vi "Field vs  IV and Ic distribution_V2.vi"() -> ()   [LabVIEW 2020]
uses:
  RT fast data.ctl
  <vilib>/LabVIEW Targets/FPGA/cRIO/shared/nicrio_ModuleControls/nicrio_cRIO-9775_RecordDataRates4ChansRing.ctl
  <vilib>/Utility/file.llb/Write Delimited Spreadsheet (DBL).vi
  global.vi
  <resource>/objmgr/ni.dex.rc
  <vilib>/Analysis/NI_AALBase.lvlib
panel:
  in  "Tab Control":enum32{"Field", "cRIO", "IV Ic Parameters"}(tab)=enum."cRIO"
  in  "Field Rate mT per sec":dbl=0.1 format="%#_13g"
  in  "Field Radius mT":dbl=10.0 format="%#_13g"
  in  "Field step mT":dbl=0.05 format="%#_13g"
  in  "Field Origin mT":dbl=-6.0 format="%#_13g"
  in  "Ramp up first T":bool=TRUE
  in  "Ramp type":string(combo)="Range"
  in  "Magnet Device Select":string(combo)="Elsa Magnet mT"
  in  "AI Channel":u8
  in  "Trigger Slope":enum8{"Positive", "Negative"}(ring)
  in  "Dist Record Samples":u32=10000
  in  "cRIO IP":string="//172.22.11.2"
  in  "Data buffer size":i32=1000
  in  "Voltage Scale factor":dbl=0.0001
  in  "Current Scale factor":dbl=1.0
  in  "IV Record Samples":u32=5000
  in  "Gate wait time us":u32=150
  in  "IV Record Data Rate":T1=200 items=["20.000 MS/s (NI 9775)"=1, "10.00 MS/s (NI 9775)"=2, "6.667 MS/s (NI 9775)"=3, "5.000 MS/s (NI 9775)"=4, "2.500 MS/s (NI 9775)"=8, "1.667 MS/s (NI 9775)"=12, "1.250 MS/s (NI 9775)"=16, "1.000 MS/s (NI 9775)"=20, "833.333 KS/s (NI 9775)"=24, "714.286 KS/s (NI 9775)"=28, "625.000 KS/s (NI 9775)"=32, "555.556 KS/s (NI 9775)"=36, "500.000 KS/s (NI 9775)"=40, "454.545 KS/s (NI 9775)"=44, "416.667 KS/s (NI 9775)"=48, "384.615 KS/s (NI 9775)"=52, "357.143 KS/s (NI 9775)"=56, "333.333 KS/s (NI 9775)"=60, "312.500 KS/s (NI 9775)"=64, "294.118 KS/s (NI 9775)"=68, "277.778 KS/s (NI 9775)"=72, "263.158 KS/s (NI 9775)"=76, "250.000 KS/s (NI 9775)"=80, "238.095 KS/s (NI 9775)"=84, "227.273 KS/s (NI 9775)"=88, "217.391 KS/s (NI 9775)"=92, "208.333 KS/s (NI 9775)"=96, "200.000 KS/s (NI 9775)"=100, "192.308 KS/s (NI 9775)"=104, "185.185 KS/s (NI 9775)"=108, "178.571 KS/s (NI 9775)"=112, "172.414 KS/s (NI 9775)"=116, "166.667 KS/s (NI 9775)"=120, "161.290 KS/s (NI 9775)"=124, "156.250 KS/s (NI 9775)"=128, "151.515 KS/s (NI 9775)"=132, "147.059 KS/s (NI 9775)"=136, "142.857 KS/s (NI 9775)"=140, "138.889 KS/s (NI 9775)"=144, "135.135 KS/s (NI 9775)"=148, "131.579 KS/s (NI 9775)"=152, "128.205 KS/s (NI 9775)"=156, "125.000 KS/s (NI 9775)"=160, "121.951 KS/s (NI 9775)"=164, "119.048 KS/s (NI 9775)"=168, "116.279 KS/s (NI 9775)"=172, "113.636 KS/s (NI 9775)"=176, "111.111 KS/s (NI 9775)"=180, "108.696 KS/s (NI 9775)"=184, "106.383 KS/s (NI 9775)"=188, "104.167 KS/s (NI 9775)"=192, "102.041 KS/s (NI 9775)"=196, "100.000 KS/s (NI 9775)"=200, "50.000 KS/s (NI 9775)"=400, "33.333 KS/s (NI 9775)"=600, "25.000 KS/s (NI 9775)"=800, "20.000 KS/s (NI 9775)"=1000, "16.667 KS/s (NI 9775)"=1200, "14.286 KS/s (NI 9775)"=1400, "12.500 KS/s (NI 9775)"=1600, "11.111 KS/s (NI 9775)"=1800, "10.000 KS/s (NI 9775)"=2000, "9.091 KS/s (NI 9775)"=2200, "8.333 KS/s (NI 9775)"=2400, "7.692 KS/s (NI 9775)"=2600, "7.143 KS/s (NI 9775)"=2800, "6.667 KS/s (NI 9775)"=3000, "6.250 KS/s (NI 9775)"=3200, "5.882 KS/s (NI 9775)"=3400, "5.556 KS/s (NI 9775)"=3600, "5.000 KS/s (NI 9775)"=4000, "4.762 KS/s (NI 9775)"=4200, "4.545 KS/s (NI 9775)"=4400, "4.348 KS/s (NI 9775)"=4600, "4.167 KS/s (NI 9775)"=4800, "4.000 KS/s (NI 9775)"=5000, "3.846 KS/s (NI 9775)"=5200, "3.571 KS/s (NI 9775)"=5600, "3.333 KS/s (NI 9775)"=6000, "3.125 KS/s (NI 9775)"=6400, "2.941 KS/s (NI 9775)"=6800, "2.778 KS/s (NI 9775)"=7200, "2.632 KS/s (NI 9775)"=7600, "2.500 KS/s (NI 9775)"=8000, "2.381 KS/s (NI 9775)"=8400, "2.273 KS/s (NI 9775)"=8800, "2.174 KS/s (NI 9775)"=9200, "2.083 KS/s (NI 9775)"=9600, "2.000 KS/s (NI 9775)"=10000, "1.923 KS/s (NI 9775)"=10400, "1.852 KS/s (NI 9775)"=10800, "1.786 KS/s (NI 9775)"=11200, "1.724 KS/s (NI 9775)"=11600, "1.667 KS/s (NI 9775)"=12000, "1.613 KS/s (NI 9775)"=12400, "1.563 KS/s (NI 9775)"=12800, "1.515 KS/s (NI 9775)"=13200, "1.471 KS/s (NI 9775)"=13600, "1.429 KS/s (NI 9775)"=14000, "1.389 KS/s (NI 9775)"=14400, "1.351 KS/s (NI 9775)"=14800, "1.316 KS/s (NI 9775)"=15200, "1.282 KS/s (NI 9775)"=15600, "1.250 KS/s (NI 9775)"=16000, "1.220 KS/s (NI 9775)"=16400, "1.190 KS/s (NI 9775)"=16800, "1.163 KS/s (NI 9775)"=17200, "1.136 KS/s (NI 9775)"=17600, "1.111 KS/s (NI 9775)"=18000, "1.087 KS/s (NI 9775)"=18400, "1.064 KS/s (NI 9775)"=18800, "1.042 KS/s (NI 9775)"=19200, "1.020 KS/s (NI 9775)"=19600, "1.000 KS/s (NI 9775)"=20000, "0.980 KS/s (NI 9775)"=20400, "0.962 KS/s (NI 9775)"=20800, "0.943 KS/s (NI 9775)"=21200, "0.926 KS/s (NI 9775)"=21600, "0.909 KS/s (NI 9775)"=22000, "0.893 KS/s (NI 9775)"=22400, "0.877 KS/s (NI 9775)"=22800, "0.862 KS/s (NI 9775)"=23200, "0.847 KS/s (NI 9775)"=23600, "0.833 KS/s (NI 9775)"=24000, "0.820 KS/s (NI 9775)"=24400, "0.806 KS/s (NI 9775)"=24800, "0.794 KS/s (NI 9775)"=25200, "0.781 KS/s (NI 9775)"=25600, "0.694 KS/s (NI 9775)"=28800, "0.625 KS/s (NI 9775)"=32000, "0.568 KS/s (NI 9775)"=35200, "0.521 KS/s (NI 9775)"=38400, "0.446 KS/s (NI 9775)"=44800, "0.391 KS/s (NI 9775)"=51200, "0.347 KS/s (NI 9775)"=57600, "0.313 KS/s (NI 9775)"=64000]
  in  "Relative threshold":dbl=0.21 format="%#_13g"
  in  "Dist Record Data Rate":T1=1 items=["20.000 MS/s (NI 9775)"=1, "10.00 MS/s (NI 9775)"=2, "6.667 MS/s (NI 9775)"=3, "5.000 MS/s (NI 9775)"=4, "2.500 MS/s (NI 9775)"=8, "1.667 MS/s (NI 9775)"=12, "1.250 MS/s (NI 9775)"=16, "1.000 MS/s (NI 9775)"=20, "833.333 KS/s (NI 9775)"=24, "714.286 KS/s (NI 9775)"=28, "625.000 KS/s (NI 9775)"=32, "555.556 KS/s (NI 9775)"=36, "500.000 KS/s (NI 9775)"=40, "454.545 KS/s (NI 9775)"=44, "416.667 KS/s (NI 9775)"=48, "384.615 KS/s (NI 9775)"=52, "357.143 KS/s (NI 9775)"=56, "333.333 KS/s (NI 9775)"=60, "312.500 KS/s (NI 9775)"=64, "294.118 KS/s (NI 9775)"=68, "277.778 KS/s (NI 9775)"=72, "263.158 KS/s (NI 9775)"=76, "250.000 KS/s (NI 9775)"=80, "238.095 KS/s (NI 9775)"=84, "227.273 KS/s (NI 9775)"=88, "217.391 KS/s (NI 9775)"=92, "208.333 KS/s (NI 9775)"=96, "200.000 KS/s (NI 9775)"=100, "192.308 KS/s (NI 9775)"=104, "185.185 KS/s (NI 9775)"=108, "178.571 KS/s (NI 9775)"=112, "172.414 KS/s (NI 9775)"=116, "166.667 KS/s (NI 9775)"=120, "161.290 KS/s (NI 9775)"=124, "156.250 KS/s (NI 9775)"=128, "151.515 KS/s (NI 9775)"=132, "147.059 KS/s (NI 9775)"=136, "142.857 KS/s (NI 9775)"=140, "138.889 KS/s (NI 9775)"=144, "135.135 KS/s (NI 9775)"=148, "131.579 KS/s (NI 9775)"=152, "128.205 KS/s (NI 9775)"=156, "125.000 KS/s (NI 9775)"=160, "121.951 KS/s (NI 9775)"=164, "119.048 KS/s (NI 9775)"=168, "116.279 KS/s (NI 9775)"=172, "113.636 KS/s (NI 9775)"=176, "111.111 KS/s (NI 9775)"=180, "108.696 KS/s (NI 9775)"=184, "106.383 KS/s (NI 9775)"=188, "104.167 KS/s (NI 9775)"=192, "102.041 KS/s (NI 9775)"=196, "100.000 KS/s (NI 9775)"=200, "50.000 KS/s (NI 9775)"=400, "33.333 KS/s (NI 9775)"=600, "25.000 KS/s (NI 9775)"=800, "20.000 KS/s (NI 9775)"=1000, "16.667 KS/s (NI 9775)"=1200, "14.286 KS/s (NI 9775)"=1400, "12.500 KS/s (NI 9775)"=1600, "11.111 KS/s (NI 9775)"=1800, "10.000 KS/s (NI 9775)"=2000, "9.091 KS/s (NI 9775)"=2200, "8.333 KS/s (NI 9775)"=2400, "7.692 KS/s (NI 9775)"=2600, "7.143 KS/s (NI 9775)"=2800, "6.667 KS/s (NI 9775)"=3000, "6.250 KS/s (NI 9775)"=3200, "5.882 KS/s (NI 9775)"=3400, "5.556 KS/s (NI 9775)"=3600, "5.000 KS/s (NI 9775)"=4000, "4.762 KS/s (NI 9775)"=4200, "4.545 KS/s (NI 9775)"=4400, "4.348 KS/s (NI 9775)"=4600, "4.167 KS/s (NI 9775)"=4800, "4.000 KS/s (NI 9775)"=5000, "3.846 KS/s (NI 9775)"=5200, "3.571 KS/s (NI 9775)"=5600, "3.333 KS/s (NI 9775)"=6000, "3.125 KS/s (NI 9775)"=6400, "2.941 KS/s (NI 9775)"=6800, "2.778 KS/s (NI 9775)"=7200, "2.632 KS/s (NI 9775)"=7600, "2.500 KS/s (NI 9775)"=8000, "2.381 KS/s (NI 9775)"=8400, "2.273 KS/s (NI 9775)"=8800, "2.174 KS/s (NI 9775)"=9200, "2.083 KS/s (NI 9775)"=9600, "2.000 KS/s (NI 9775)"=10000, "1.923 KS/s (NI 9775)"=10400, "1.852 KS/s (NI 9775)"=10800, "1.786 KS/s (NI 9775)"=11200, "1.724 KS/s (NI 9775)"=11600, "1.667 KS/s (NI 9775)"=12000, "1.613 KS/s (NI 9775)"=12400, "1.563 KS/s (NI 9775)"=12800, "1.515 KS/s (NI 9775)"=13200, "1.471 KS/s (NI 9775)"=13600, "1.429 KS/s (NI 9775)"=14000, "1.389 KS/s (NI 9775)"=14400, "1.351 KS/s (NI 9775)"=14800, "1.316 KS/s (NI 9775)"=15200, "1.282 KS/s (NI 9775)"=15600, "1.250 KS/s (NI 9775)"=16000, "1.220 KS/s (NI 9775)"=16400, "1.190 KS/s (NI 9775)"=16800, "1.163 KS/s (NI 9775)"=17200, "1.136 KS/s (NI 9775)"=17600, "1.111 KS/s (NI 9775)"=18000, "1.087 KS/s (NI 9775)"=18400, "1.064 KS/s (NI 9775)"=18800, "1.042 KS/s (NI 9775)"=19200, "1.020 KS/s (NI 9775)"=19600, "1.000 KS/s (NI 9775)"=20000, "0.980 KS/s (NI 9775)"=20400, "0.962 KS/s (NI 9775)"=20800, "0.943 KS/s (NI 9775)"=21200, "0.926 KS/s (NI 9775)"=21600, "0.909 KS/s (NI 9775)"=22000, "0.893 KS/s (NI 9775)"=22400, "0.877 KS/s (NI 9775)"=22800, "0.862 KS/s (NI 9775)"=23200, "0.847 KS/s (NI 9775)"=23600, "0.833 KS/s (NI 9775)"=24000, "0.820 KS/s (NI 9775)"=24400, "0.806 KS/s (NI 9775)"=24800, "0.794 KS/s (NI 9775)"=25200, "0.781 KS/s (NI 9775)"=25600, "0.694 KS/s (NI 9775)"=28800, "0.625 KS/s (NI 9775)"=32000, "0.568 KS/s (NI 9775)"=35200, "0.521 KS/s (NI 9775)"=38400, "0.446 KS/s (NI 9775)"=44800, "0.391 KS/s (NI 9775)"=51200, "0.347 KS/s (NI 9775)"=57600, "0.313 KS/s (NI 9775)"=64000]
  in  "Zero avg":i32=500
  in  "Count ms half of T":u32=15
  in  "Wait before trigger us":u32=10100
  in  "Tab Control 2":enum32{"IV", "Ic"}(tab)
  out "IV parameters":T2={"Records Num"=1, "AI Trigger Configuration"={"Trigger Slope"=enum."Positive", "Trigger Level"=0.10009765625, "Hystesis Value"=0.094970703125, "AI Channel"=0}, "Record PreTrigger Samples"=1, "Record Samples"=5000, "Ic Cut off or curve"=FALSE, "Gate wait time us"=150, "Record Data Rate"=200, "Count ms half of T"=15, "Wait before trigger us"=10100} {"Record Data Rate" items=["20.000 MS/s (NI 9775)"=1, "10.00 MS/s (NI 9775)"=2, "6.667 MS/s (NI 9775)"=3, "5.000 MS/s (NI 9775)"=4, "2.500 MS/s (NI 9775)"=8, "1.667 MS/s (NI 9775)"=12, "1.250 MS/s (NI 9775)"=16, "1.000 MS/s (NI 9775)"=20, "833.333 KS/s (NI 9775)"=24, "714.286 KS/s (NI 9775)"=28, "625.000 KS/s (NI 9775)"=32, "555.556 KS/s (NI 9775)"=36, "500.000 KS/s (NI 9775)"=40, "454.545 KS/s (NI 9775)"=44, "416.667 KS/s (NI 9775)"=48, "384.615 KS/s (NI 9775)"=52, "357.143 KS/s (NI 9775)"=56, "333.333 KS/s (NI 9775)"=60, "312.500 KS/s (NI 9775)"=64, "294.118 KS/s (NI 9775)"=68, "277.778 KS/s (NI 9775)"=72, "263.158 KS/s (NI 9775)"=76, "250.000 KS/s (NI 9775)"=80, "238.095 KS/s (NI 9775)"=84, "227.273 KS/s (NI 9775)"=88, "217.391 KS/s (NI 9775)"=92, "208.333 KS/s (NI 9775)"=96, "200.000 KS/s (NI 9775)"=100, "192.308 KS/s (NI 9775)"=104, "185.185 KS/s (NI 9775)"=108, "178.571 KS/s (NI 9775)"=112, "172.414 KS/s (NI 9775)"=116, "166.667 KS/s (NI 9775)"=120, "161.290 KS/s (NI 9775)"=124, "156.250 KS/s (NI 9775)"=128, "151.515 KS/s (NI 9775)"=132, "147.059 KS/s (NI 9775)"=136, "142.857 KS/s (NI 9775)"=140, "138.889 KS/s (NI 9775)"=144, "135.135 KS/s (NI 9775)"=148, "131.579 KS/s (NI 9775)"=152, "128.205 KS/s (NI 9775)"=156, "125.000 KS/s (NI 9775)"=160, "121.951 KS/s (NI 9775)"=164, "119.048 KS/s (NI 9775)"=168, "116.279 KS/s (NI 9775)"=172, "113.636 KS/s (NI 9775)"=176, "111.111 KS/s (NI 9775)"=180, "108.696 KS/s (NI 9775)"=184, "106.383 KS/s (NI 9775)"=188, "104.167 KS/s (NI 9775)"=192, "102.041 KS/s (NI 9775)"=196, "100.000 KS/s (NI 9775)"=200, "50.000 KS/s (NI 9775)"=400, "33.333 KS/s (NI 9775)"=600, "25.000 KS/s (NI 9775)"=800, "20.000 KS/s (NI 9775)"=1000, "16.667 KS/s (NI 9775)"=1200, "14.286 KS/s (NI 9775)"=1400, "12.500 KS/s (NI 9775)"=1600, "11.111 KS/s (NI 9775)"=1800, "10.000 KS/s (NI 9775)"=2000, "9.091 KS/s (NI 9775)"=2200, "8.333 KS/s (NI 9775)"=2400, "7.692 KS/s (NI 9775)"=2600, "7.143 KS/s (NI 9775)"=2800, "6.667 KS/s (NI 9775)"=3000, "6.250 KS/s (NI 9775)"=3200, "5.882 KS/s (NI 9775)"=3400, "5.556 KS/s (NI 9775)"=3600, "5.000 KS/s (NI 9775)"=4000, "4.762 KS/s (NI 9775)"=4200, "4.545 KS/s (NI 9775)"=4400, "4.348 KS/s (NI 9775)"=4600, "4.167 KS/s (NI 9775)"=4800, "4.000 KS/s (NI 9775)"=5000, "3.846 KS/s (NI 9775)"=5200, "3.571 KS/s (NI 9775)"=5600, "3.333 KS/s (NI 9775)"=6000, "3.125 KS/s (NI 9775)"=6400, "2.941 KS/s (NI 9775)"=6800, "2.778 KS/s (NI 9775)"=7200, "2.632 KS/s (NI 9775)"=7600, "2.500 KS/s (NI 9775)"=8000, "2.381 KS/s (NI 9775)"=8400, "2.273 KS/s (NI 9775)"=8800, "2.174 KS/s (NI 9775)"=9200, "2.083 KS/s (NI 9775)"=9600, "2.000 KS/s (NI 9775)"=10000, "1.923 KS/s (NI 9775)"=10400, "1.852 KS/s (NI 9775)"=10800, "1.786 KS/s (NI 9775)"=11200, "1.724 KS/s (NI 9775)"=11600, "1.667 KS/s (NI 9775)"=12000, "1.613 KS/s (NI 9775)"=12400, "1.563 KS/s (NI 9775)"=12800, "1.515 KS/s (NI 9775)"=13200, "1.471 KS/s (NI 9775)"=13600, "1.429 KS/s (NI 9775)"=14000, "1.389 KS/s (NI 9775)"=14400, "1.351 KS/s (NI 9775)"=14800, "1.316 KS/s (NI 9775)"=15200, "1.282 KS/s (NI 9775)"=15600, "1.250 KS/s (NI 9775)"=16000, "1.220 KS/s (NI 9775)"=16400, "1.190 KS/s (NI 9775)"=16800, "1.163 KS/s (NI 9775)"=17200, "1.136 KS/s (NI 9775)"=17600, "1.111 KS/s (NI 9775)"=18000, "1.087 KS/s (NI 9775)"=18400, "1.064 KS/s (NI 9775)"=18800, "1.042 KS/s (NI 9775)"=19200, "1.020 KS/s (NI 9775)"=19600, "1.000 KS/s (NI 9775)"=20000, "0.980 KS/s (NI 9775)"=20400, "0.962 KS/s (NI 9775)"=20800, "0.943 KS/s (NI 9775)"=21200, "0.926 KS/s (NI 9775)"=21600, "0.909 KS/s (NI 9775)"=22000, "0.893 KS/s (NI 9775)"=22400, "0.877 KS/s (NI 9775)"=22800, "0.862 KS/s (NI 9775)"=23200, "0.847 KS/s (NI 9775)"=23600, "0.833 KS/s (NI 9775)"=24000, "0.820 KS/s (NI 9775)"=24400, "0.806 KS/s (NI 9775)"=24800, "0.794 KS/s (NI 9775)"=25200, "0.781 KS/s (NI 9775)"=25600, "0.694 KS/s (NI 9775)"=28800, "0.625 KS/s (NI 9775)"=32000, "0.568 KS/s (NI 9775)"=35200, "0.521 KS/s (NI 9775)"=38400, "0.446 KS/s (NI 9775)"=44800, "0.391 KS/s (NI 9775)"=51200, "0.347 KS/s (NI 9775)"=57600, "0.313 KS/s (NI 9775)"=64000]}
  out "Ic parameters":T2={"Records Num"=10000, "AI Trigger Configuration"={"Trigger Slope"=enum."Positive", "Trigger Level"=0.2392578125, "Hystesis Value"=0.0, "AI Channel"=0}, "Record PreTrigger Samples"=1, "Record Samples"=16, "Ic Cut off or curve"=TRUE, "Gate wait time us"=150, "Record Data Rate"=1, "Count ms half of T"=15, "Wait before trigger us"=10100} {"Record Data Rate" items=["20.000 MS/s (NI 9775)"=1, "10.00 MS/s (NI 9775)"=2, "6.667 MS/s (NI 9775)"=3, "5.000 MS/s (NI 9775)"=4, "2.500 MS/s (NI 9775)"=8, "1.667 MS/s (NI 9775)"=12, "1.250 MS/s (NI 9775)"=16, "1.000 MS/s (NI 9775)"=20, "833.333 KS/s (NI 9775)"=24, "714.286 KS/s (NI 9775)"=28, "625.000 KS/s (NI 9775)"=32, "555.556 KS/s (NI 9775)"=36, "500.000 KS/s (NI 9775)"=40, "454.545 KS/s (NI 9775)"=44, "416.667 KS/s (NI 9775)"=48, "384.615 KS/s (NI 9775)"=52, "357.143 KS/s (NI 9775)"=56, "333.333 KS/s (NI 9775)"=60, "312.500 KS/s (NI 9775)"=64, "294.118 KS/s (NI 9775)"=68, "277.778 KS/s (NI 9775)"=72, "263.158 KS/s (NI 9775)"=76, "250.000 KS/s (NI 9775)"=80, "238.095 KS/s (NI 9775)"=84, "227.273 KS/s (NI 9775)"=88, "217.391 KS/s (NI 9775)"=92, "208.333 KS/s (NI 9775)"=96, "200.000 KS/s (NI 9775)"=100, "192.308 KS/s (NI 9775)"=104, "185.185 KS/s (NI 9775)"=108, "178.571 KS/s (NI 9775)"=112, "172.414 KS/s (NI 9775)"=116, "166.667 KS/s (NI 9775)"=120, "161.290 KS/s (NI 9775)"=124, "156.250 KS/s (NI 9775)"=128, "151.515 KS/s (NI 9775)"=132, "147.059 KS/s (NI 9775)"=136, "142.857 KS/s (NI 9775)"=140, "138.889 KS/s (NI 9775)"=144, "135.135 KS/s (NI 9775)"=148, "131.579 KS/s (NI 9775)"=152, "128.205 KS/s (NI 9775)"=156, "125.000 KS/s (NI 9775)"=160, "121.951 KS/s (NI 9775)"=164, "119.048 KS/s (NI 9775)"=168, "116.279 KS/s (NI 9775)"=172, "113.636 KS/s (NI 9775)"=176, "111.111 KS/s (NI 9775)"=180, "108.696 KS/s (NI 9775)"=184, "106.383 KS/s (NI 9775)"=188, "104.167 KS/s (NI 9775)"=192, "102.041 KS/s (NI 9775)"=196, "100.000 KS/s (NI 9775)"=200, "50.000 KS/s (NI 9775)"=400, "33.333 KS/s (NI 9775)"=600, "25.000 KS/s (NI 9775)"=800, "20.000 KS/s (NI 9775)"=1000, "16.667 KS/s (NI 9775)"=1200, "14.286 KS/s (NI 9775)"=1400, "12.500 KS/s (NI 9775)"=1600, "11.111 KS/s (NI 9775)"=1800, "10.000 KS/s (NI 9775)"=2000, "9.091 KS/s (NI 9775)"=2200, "8.333 KS/s (NI 9775)"=2400, "7.692 KS/s (NI 9775)"=2600, "7.143 KS/s (NI 9775)"=2800, "6.667 KS/s (NI 9775)"=3000, "6.250 KS/s (NI 9775)"=3200, "5.882 KS/s (NI 9775)"=3400, "5.556 KS/s (NI 9775)"=3600, "5.000 KS/s (NI 9775)"=4000, "4.762 KS/s (NI 9775)"=4200, "4.545 KS/s (NI 9775)"=4400, "4.348 KS/s (NI 9775)"=4600, "4.167 KS/s (NI 9775)"=4800, "4.000 KS/s (NI 9775)"=5000, "3.846 KS/s (NI 9775)"=5200, "3.571 KS/s (NI 9775)"=5600, "3.333 KS/s (NI 9775)"=6000, "3.125 KS/s (NI 9775)"=6400, "2.941 KS/s (NI 9775)"=6800, "2.778 KS/s (NI 9775)"=7200, "2.632 KS/s (NI 9775)"=7600, "2.500 KS/s (NI 9775)"=8000, "2.381 KS/s (NI 9775)"=8400, "2.273 KS/s (NI 9775)"=8800, "2.174 KS/s (NI 9775)"=9200, "2.083 KS/s (NI 9775)"=9600, "2.000 KS/s (NI 9775)"=10000, "1.923 KS/s (NI 9775)"=10400, "1.852 KS/s (NI 9775)"=10800, "1.786 KS/s (NI 9775)"=11200, "1.724 KS/s (NI 9775)"=11600, "1.667 KS/s (NI 9775)"=12000, "1.613 KS/s (NI 9775)"=12400, "1.563 KS/s (NI 9775)"=12800, "1.515 KS/s (NI 9775)"=13200, "1.471 KS/s (NI 9775)"=13600, "1.429 KS/s (NI 9775)"=14000, "1.389 KS/s (NI 9775)"=14400, "1.351 KS/s (NI 9775)"=14800, "1.316 KS/s (NI 9775)"=15200, "1.282 KS/s (NI 9775)"=15600, "1.250 KS/s (NI 9775)"=16000, "1.220 KS/s (NI 9775)"=16400, "1.190 KS/s (NI 9775)"=16800, "1.163 KS/s (NI 9775)"=17200, "1.136 KS/s (NI 9775)"=17600, "1.111 KS/s (NI 9775)"=18000, "1.087 KS/s (NI 9775)"=18400, "1.064 KS/s (NI 9775)"=18800, "1.042 KS/s (NI 9775)"=19200, "1.020 KS/s (NI 9775)"=19600, "1.000 KS/s (NI 9775)"=20000, "0.980 KS/s (NI 9775)"=20400, "0.962 KS/s (NI 9775)"=20800, "0.943 KS/s (NI 9775)"=21200, "0.926 KS/s (NI 9775)"=21600, "0.909 KS/s (NI 9775)"=22000, "0.893 KS/s (NI 9775)"=22400, "0.877 KS/s (NI 9775)"=22800, "0.862 KS/s (NI 9775)"=23200, "0.847 KS/s (NI 9775)"=23600, "0.833 KS/s (NI 9775)"=24000, "0.820 KS/s (NI 9775)"=24400, "0.806 KS/s (NI 9775)"=24800, "0.794 KS/s (NI 9775)"=25200, "0.781 KS/s (NI 9775)"=25600, "0.694 KS/s (NI 9775)"=28800, "0.625 KS/s (NI 9775)"=32000, "0.568 KS/s (NI 9775)"=35200, "0.521 KS/s (NI 9775)"=38400, "0.446 KS/s (NI 9775)"=44800, "0.391 KS/s (NI 9775)"=51200, "0.347 KS/s (NI 9775)"=57600, "0.313 KS/s (NI 9775)"=64000]}
  out "Threshold":dbl=0.23925537109375
  in  "Stop loop":bool
  out "Current Field mT":dbl=4.0
  in  "Name":string="book714"
  in  "Contour plot folder":path=path "C:/Users/gyue/Desktop/Data folder 20210604"
  out "Histogram Graph":T3(graph)={"X Values"=[0.071759033203125, 0.08246459960937501, 0.09317016601562501, 0.10387573242187502, 0.11458129882812502, 0.12528686523437502, 0.13599243164062502, 0.14669799804687503, 0.15740356445312503, 0.16810913085937504, 0.17881469726562504, 0.18952026367187505, 0.20022583007812506, 0.21093139648437506, 0.22163696289062507, 0.23234252929687507, 0.24304809570312508, 0.25375366210937506, 0.26445922851562503, 0.275164794921875, 0.285870361328125, 0.29657592773437497, 0.30728149414062494, 0.3179870605468749, 0.3286926269531249, 0.3393981933593749, 0.35010375976562486, 0.36080932617187483, 0.3715148925781248, 0.3822204589843748, 0.39292602539062477, 0.40363159179687474, 0.4143371582031247, 0.4250427246093747, 0.4357482910156247, 0.44645385742187466, 0.45715942382812463, 0.4678649902343746, 0.4785705566406246, 0.48927612304687457, 0.49998168945312454, 0.5106872558593746, 0.5213928222656246, 0.5320983886718745, 0.5428039550781245, 0.5535095214843745, 0.5642150878906245, 0.5749206542968744, 0.5856262207031244, 0.5963317871093744, 0.6070373535156244, 0.6177429199218744, 0.6284484863281243, 0.6391540527343743, 0.6498596191406243, 0.6605651855468743, 0.6712707519531242, 0.6819763183593742, 0.6926818847656242, 0.7033874511718742, 0.7140930175781242, 0.7247985839843741, 0.7355041503906241, 0.7462097167968741, 0.7569152832031241, 0.767620849609374, 0.778326416015624, 0.789031982421874, 0.799737548828124, 0.810443115234374, 0.8211486816406239, 0.8318542480468739, 0.8425598144531239, 0.8532653808593739, 0.8639709472656238, 0.8746765136718738, 0.8853820800781238, 0.8960876464843738, 0.9067932128906238, 0.9174987792968737, 0.9282043457031237, 0.9389099121093737, 0.9496154785156237, 0.9603210449218736, 0.9710266113281236, 0.9817321777343736, 0.9924377441406236, 1.0031433105468737, 1.0138488769531238, 1.0245544433593738, 1.035260009765624, 1.045965576171874, 1.0566711425781241, 1.0673767089843742, 1.0780822753906243, 1.0887878417968744, 1.0994934082031245, 1.1101989746093746, 1.1209045410156246, 1.1316101074218747], "Histogram: h(x)"=[3, 7, 26, 37, 47, 48, 55, 30, 43, 66, 43, 44, 49, 47, 73, 50, 50, 44, 36, 30, 51, 45, 51, 53, 41, 42, 27, 32, 27, 30, 25, 34, 32, 31, 30, 36, 24, 24, 23, 27, 42, 34, 32, 35, 33, 31, 40, 35, 46, 30, 37, 36, 32, 23, 28, 21, 18, 22, 35, 35, 20, 37, 57, 50, 68, 76, 87, 140, 206, 207, 275, 352, 431, 446, 556, 598, 536, 514, 558, 482, 401, 411, 336, 269, 177, 158, 137, 82, 52, 54, 23, 19, 10, 7, 4, 2, 0, 2, 1, 1]}
  out "IV curve":cluster{"Y":dbl[], "Y":dbl[]}[](graph)
  out "error out":errorcluster
  # "Voltage x factor=uA"
  # "Voltage x factor=V"
  # "IV setting"
  # "Distribution setting"
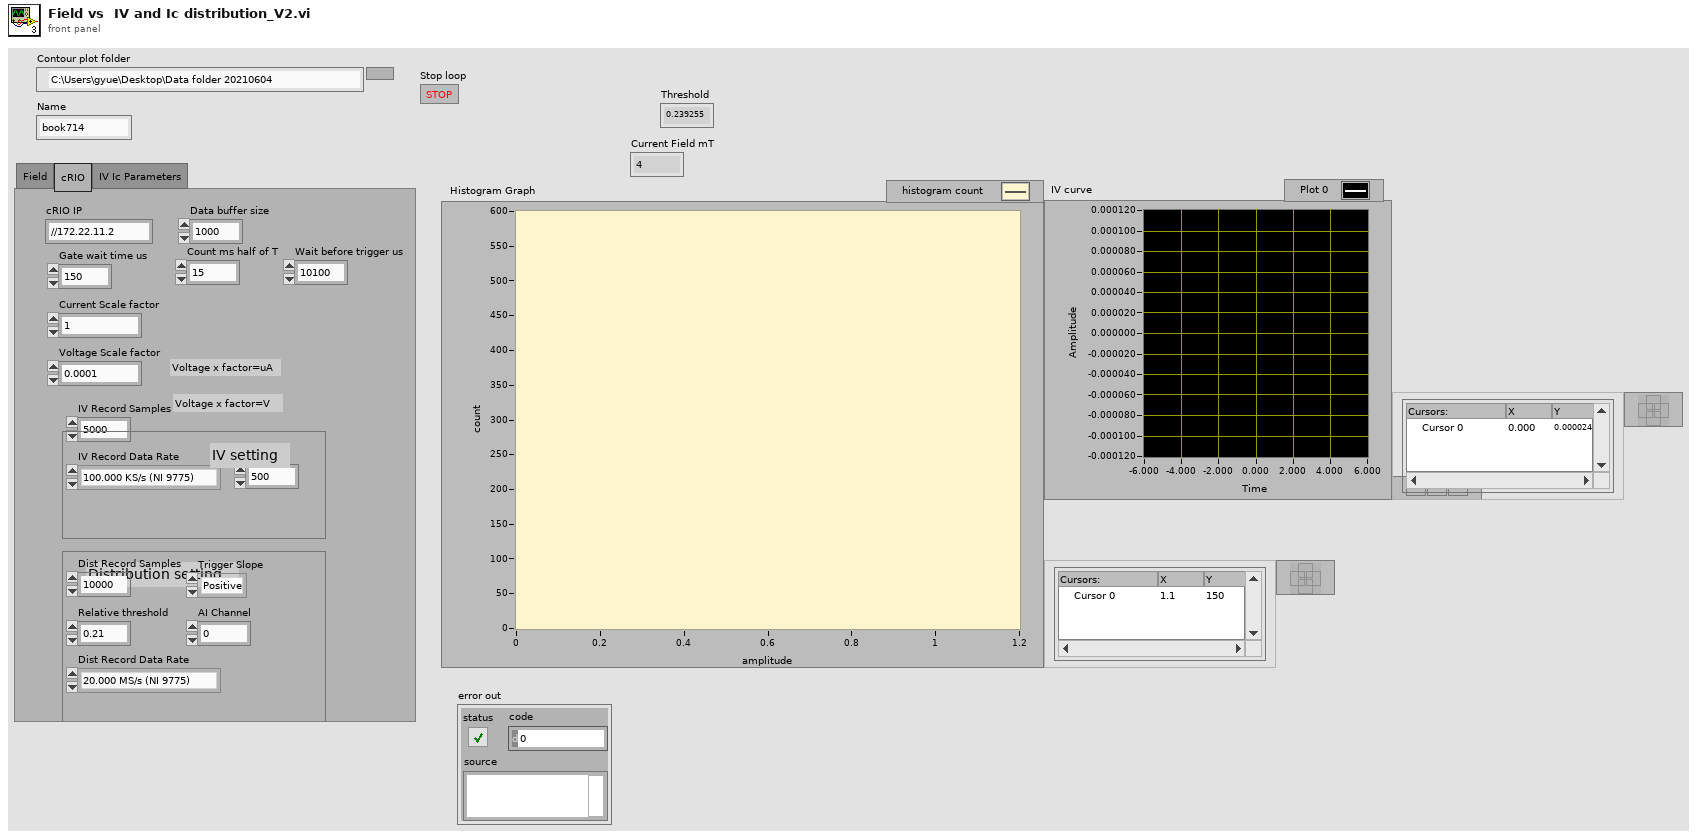
[diagram p1: front panel]
types:
  T1 = typedef "nicrio_cRIO-9775_RecordDataRates4ChansRing.ctl" = u16
  T2 = typedef "RT fast data.ctl" = cluster{"Records Num":i32, "AI Trigger Configuration":cluster{"Trigger Slope":enum8{"Positive", "Negative"}, "Trigger Level":fxp<+/-,17,5>, "Hystesis Value":fxp<+,16,4>, "AI Channel":u8}, "Record PreTrigger Samples":u32, "Record Samples":u32, "Ic Cut off or curve":bool, "Gate wait time us":u32, "Record Data Rate":T1, "Count ms half of T":u32, "Wait before trigger us":u32}
  T3 = cluster{"X Values":dbl[], "Histogram: h(x)":i32[]}
  T4 = cluster{"Trigger Slope":enum8{"Positive", "Negative"}, "Trigger Level":fxp<+/-,17,5>, "Hystesis Value":fxp<+,16,4>, "AI Channel":u8}
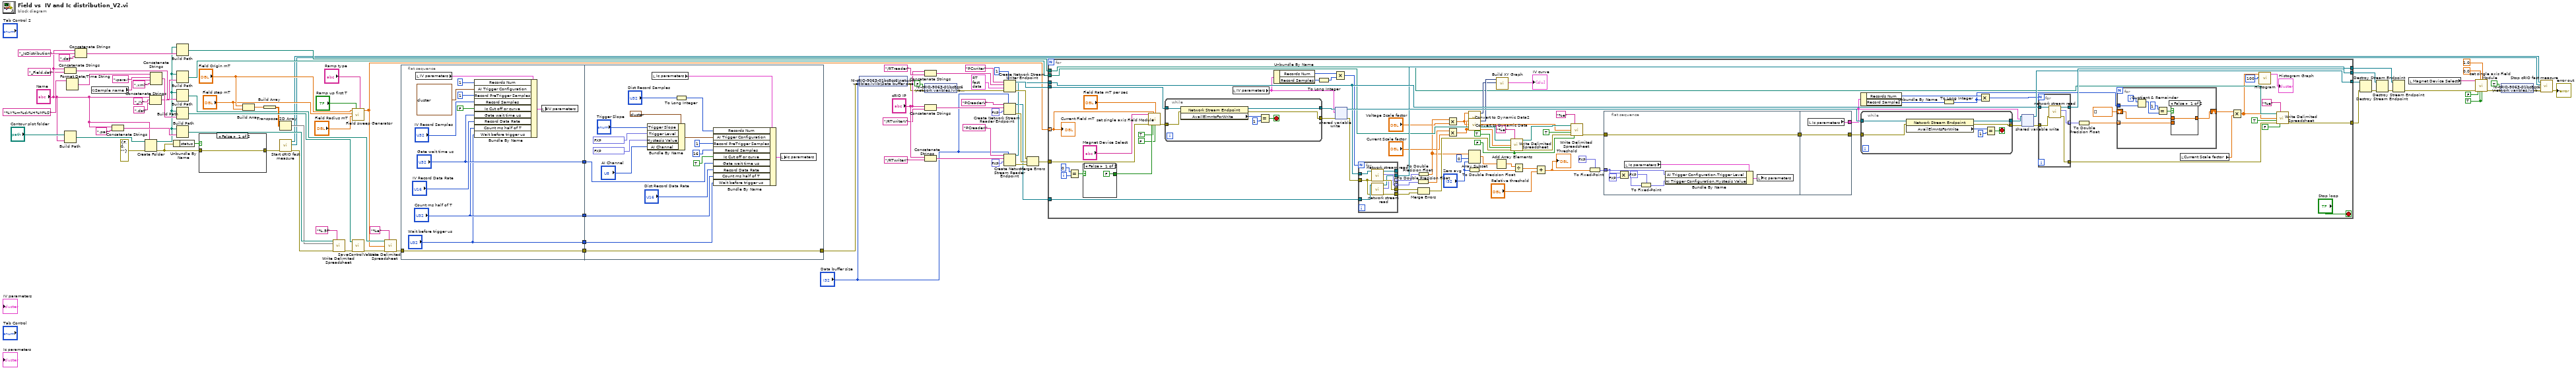
[diagram p0: block diagram]
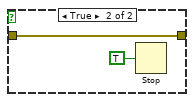
[diagram p2: hidden frame]
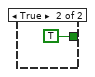
[diagram p3: hidden frame]
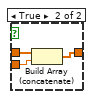
[diagram p4: hidden frame]
diagram:
  w11 = TRUE ("final")
  n1 = Concatenate Strings("Name", "_Field.dat" ("string")) -> (w29:string)
  n2 = Build Path(base path="Contour plot folder", name or relative path="Name") -> (appended path=w47:path)
  n3 = Format Date/Time String(time format string (%c)="%Y%m%d-%H%M%S") -> (date/time string=w43:string)  [unwired: 2 in]
  n4 = Concatenate Strings("Name", "_IcDistribution" ("string"), ".dat" ("string")) -> (w36:string)
  n5 = global read "global.vi" "Sample name"() -> (w42:string)
  n6 = Concatenate Strings("Name", ".par" ("string")) -> (w54:string)
  n7 = Create Folder(prompt (Create Folder)="Name", path (use dialog)=w47, error in=errorcluster {"status"=FALSE, "code"=0, "source"=""}) -> (created path=w28:path, error out=w44:errorcluster)  [unwired: 1 out]
  n8 = Concatenate Strings("Name", "_IV" ("string"), ".dat" ("string")) -> (w48:string)
  n9 = Concatenate Strings(w43, "-para-" ("string"), w42, ".xml" ("string")) -> (w58:string)
  n10 = Unbundle By Name(w44) -> ("status"=w45:bool)
  n11 = Build Path(base path=w28, name or relative path=w36) -> (appended path=w34:path)
  n12 = Build Path(base path=w28, name or relative path=w48) -> (appended path=w35:path)
  n13 = Build Path(base path=w28, name or relative path=w29) -> (appended path=w27:path)
  n14 = Build Path(base path=w28, name or relative path=w58) -> (appended path=w56:path)
  n15 = Build Path(base path=w28, name or relative path=w54) -> (appended path=w53:path)
  n16 = case shown="False" w45 {
    tunnel: [w93 w95] -> w8
    tunnel: w44 -> [w93 w95]
    frame False {
    }
    frame True {
      n17 = Stop(stop? (T)=TRUE) -> ()
    }
  }
  n18 = Build Array("Field Origin mT", "Field step mT") -> (w51:dbl[])
  n19 = Build Array(w51) -> (w50:dbl[][])
  n20 = Transpose 2D Array(2D array=w50) -> (transposed array=w49:dbl[][])
  n21 = call "Start cRIO fast measure.vi"("error in (no error)"=w8) -> ("error out"=w7:errorcluster, "vi reference"=w3:refnum<vi>, "application reference"=w4:refnum<vi>)  [unwired: 8 in]
  n22 = call-poly <vilib>:"Write Delimited Spreadsheet.vi"("file path (dialog if empty)"=w53, "format (%.3f)"="%.5f", "2D data"=w49, "error in (no error)"=w7) -> ("error out"=w46:errorcluster)  [unwired: 10 in, 1 out]
  n23 = call "Field sweep Generator.vi"("Ramp type"="Ramp type", "Ramp up first T"="Ramp up first T", "Field Radius"="Field Radius mT", "Field step"="Field step mT", "Field Origin"="Field Origin mT") -> ("output array"=w20:dbl[])  [unwired: 6 in]
  n24 = call "SaveControlValues.vi"("XML File Path"=w56, "error in (no error)"=w46) -> ("error out"=w25:errorcluster)  [unwired: 8 in]
  n25 = call-poly <vilib>:"Write Delimited Spreadsheet.vi"("file path (dialog if empty)"=w27, "format (%.3f)"="%e", "1D data"=w20, "error in (no error)"=w25) -> ("error out"=w24:errorcluster)  [unwired: 10 in, 1 out]
  n26 = flat-sequence {
    tunnel: w24 -> [w107]
    tunnel: [w107] -> w22
    tunnel: ["Gate wait time us"] -> w21
    tunnel: ["Count ms half of T"] -> w6
    tunnel: ["Wait before trigger us"] -> w5
    tunnel: [w125] -> w23
    tunnel: w22 -> [w125]
    tunnel: w21 -> [w117]
    tunnel: w6 -> [w109]
    tunnel: w5 -> [w108]
    frame #0 {
      n27 = local read "IV parameters"() -> (w106:T2)
      n28 = Bundle By Name(cluster=w106, "Records Num"=1, "AI Trigger Configuration"=T4 {"Trigger Slope"=enum."Positive", "Trigger Level"=0.10009765625, "Hystesis Value"=0.094970703125, "AI Channel"=0}, "Record PreTrigger Samples"=u32 1, "Record Samples"="IV Record Samples", "Ic Cut off or curve"=FALSE, "Gate wait time us"="Gate wait time us", "Record Data Rate"="IV Record Data Rate", "Count ms half of T"="Count ms half of T", "Wait before trigger us"="Wait before trigger us") -> (w98:T2)
      n29 = local write "IV parameters"(w98) -> ()
    }
    frame #1 {
      n30 = Bundle By Name(cluster=T4 {"Trigger Slope"=enum."Positive", "Trigger Level"=0.1708984375, "Hystesis Value"=0.162353515625, "AI Channel"=0} ("AI Trigger Configuration"), "Trigger Slope"="Trigger Slope", "Trigger Level"=fxp<+/-,17,5> 0.14990234375, "Hystesis Value"=fxp<+,16,4> 0.10009765625, "AI Channel"="AI Channel") -> (w113:T4)
      n31 = local read "Ic parameters"() -> (w124:T2)
      n32 = To Long Integer(number="Dist Record Samples") -> (32bit integer=w122:i32)
      n33 = Bundle By Name(cluster=w124, "Records Num"=w122, "AI Trigger Configuration"=w113, "Record PreTrigger Samples"=u32 1, "Record Samples"=u32 16, "Ic Cut off or curve"=TRUE, "Gate wait time us"=w117, "Record Data Rate"="Dist Record Data Rate", "Count ms half of T"=w109, "Wait before trigger us"=w108) -> (w112:T2)
      n34 = local write "Ic parameters"(w112) -> ()
    }
  }
  n35 = shared-variable "NI-cRIO-9063-01bc8cc6\\network varibles.lvlib\\Data buffer size"("Data buffer size", error in=w23) -> (error out=w71:errorcluster)
  n36 = shared-variable "NI-cRIO-9063-01bc8cc6\\network varibles.lvlib\\RT Stop"(FALSE ("RT Stop"), error in=w71) -> (error out=w78:errorcluster)
  n37 = Concatenate Strings("cRIO IP", "/RTreader" ("string")) -> (w88:string)
  n38 = Concatenate Strings("cRIO IP", "/RTwriterV" ("string")) -> (w80:string)
  n39 = Concatenate Strings("cRIO IP", "/RTwriterI" ("string")) -> (w73:string)
  n40 = Create Network Stream Writer Endpoint(7:1 ("writer buffer size"), 8:w78, 9:T2 {"Records Num"=0, "AI Trigger Configuration"={"Trigger Slope"=enum."Positive", "Trigger Level"=0.0, "Hystesis Value"=0.0, "AI Channel"=0}, "Record PreTrigger Samples"=0, "Record Samples"=0, "Ic Cut off or curve"=FALSE, "Gate wait time us"=0, "Record Data Rate"=1, "Count ms half of T"=15, "Wait before trigger us"=10100} ("Parameters 4"), 10:w88, 11:"PCwriter" ("writer name")) -> (0:w86:errorcluster, 3:w85:refnum<k21>)  [unwired: 2 in]
  n41 = Create Network Stream Reader Endpoint(7:"Data buffer size", 9:fxp<+/-,17,5> 0.0, 10:w80, 11:"PCreaderV" ("reader name")) -> (0:w77:errorcluster, 3:w65:refnum<k21>)  [unwired: 3 in]
  n42 = Create Network Stream Reader Endpoint(7:"Data buffer size", 9:fxp<+/-,17,5> 0.0, 10:w73, 11:"PCreaderI" ("reader name")) -> (0:w70:errorcluster, 3:w68:refnum<k21>)  [unwired: 3 in]
  n43 = Merge Errors(w86, w77, w70) -> (w84:errorcluster)
  n44 = for {
    tunnel: w85 -> [w208]
    tunnel: [w197] -> w66
    tunnel: w84 -> [w138]
    tunnel: [w165] -> w63
    tunnel: w68 -> [w202]
    tunnel: [w200] -> w67
    tunnel: w65 -> [w186]
    tunnel: [w185] -> w64
    tunnel: w35 -> [w171]
    tunnel: w34 -> [w163]
    tunnel: w20 -> [w136] mode=indexing
    i -> [w132]
    stop <- "Stop loop" stop-if-true
    w149 = FALSE ("transpose? (no:F)")
    n45 = Equal?(x=0, y=w132) -> (x = y?=w130:bool)
    n46 = case shown="False" w130 {
      tunnel: [FALSE ("Init") TRUE ("Init")] -> w129
      frame False {
      }
      frame True {
      }
    }
    n47 = call "set single axis Field Module.vi"("Magnet Device Select"="Magnet Device Select", "error in (no error)"=w138, "Init"=w129, "Field Target mT"=w136, "Exec"=TRUE, "Field Rate mT per sec"="Field Rate mT per sec", "final"=FALSE) -> ("error out"=w137:errorcluster)  [unwired: 12 in]
    n48 = while {
      tunnel: w208 -> [w261]
      tunnel: w137 -> [w260]
      tunnel: [w256] -> w209
      tunnel: [w255] -> w207
      stop <- w257 stop-if-true
      n49 = property class="Network Stream Endpoint"(reference=w261, error in=w260) -> (reference out=w256:refnum<k21>, error out=w255:errorcluster, "AvailElmntsForWrite"=w259:i32)
      n50 = Equal?(x=w259, y=1) -> (x = y?=w257:bool)
    }
    n51 = local read "IV parameters"() -> (w191:T2)
    n52 = Unbundle By Name(w191) -> ("Records Num"=w190:i32, "Record Samples"=w189:u32)
    n53 = To Long Integer(number=w189) -> (32bit integer=w188:i32)
    n54 = Multiply(x=w190, y=w188) -> (x*y=w187:i32)
    n55 = shared-variable-write(w209, w207, w191) -> (w205:refnum<k21>, w206:errorcluster)  [unwired: 1 in, 1 out]
    n56 = for {
      N: w187 -> [_]
      tunnel: w202 -> [w254]
      tunnel: w206 -> [w247]
      tunnel: [w253] -> w170 mode=indexing
      tunnel: [w252] -> _
      tunnel: [w251] -> w184
      tunnel: w186 -> [w250]
      tunnel: [w249] -> w185
      tunnel: [w248] -> w169 mode=indexing
      tunnel: [w246] -> w183
      n57 = call "network stream read.vi"("error in (no error)"=w247, "endpoint in"=w254) -> ("error out"=w251:errorcluster, "Data"=w253:fxp<+/-,17,5>, "endpoint out"=w252:refnum<k21>)  [unwired: 7 in]
      n58 = call "network stream read.vi"("error in (no error)"=w247, "endpoint in"=w250) -> ("error out"=w246:errorcluster, "Data"=w248:fxp<+/-,17,5>, "endpoint out"=w249:refnum<k21>)  [unwired: 7 in]
    }
    n59 = To Double Precision Float(number=w170) -> (double precision float=w148:dbl[])
    n60 = Merge Errors(w184, w183) -> (w176:errorcluster)
    n61 = To Double Precision Float(number=w169) -> (double precision float=w145:dbl[])
    n62 = Multiply(x=w145, y="Voltage Scale factor") -> (x*y=w143:dbl[])
    n63 = Multiply(x=w148, y="Current Scale factor") -> (x*y=w146:dbl[])
    n64 = call "Convert to Dynamic Data2"("Array"=w143) -> ("Dynamic Data Type"=w195:dynamicdata)  [unwired: 3 in]
    n65 = call "Convert to Dynamic Data"("Array"=w146) -> ("Dynamic Data Type"=w196:dynamicdata)  [unwired: 3 in]
    n66 = Array Subset(array=w145, index=0, length="Zero avg") -> (w160:dbl[])
    n67 = To Double Precision Float(number="Zero avg") -> (double precision float=w157:dbl)
    n68 = Add Array Elements(numeric array=w160) -> (sum=w159:dbl)
    n69 = call "Build XY Graph"("Y Input"=w195, "X Input"=w196) -> ("XY Graph"=→"IV curve":cluster{"X":dbl[], "Y":dbl[]}[])  [unwired: 8 in, 1 out]
    n70 = call-poly <vilib>:"Write Delimited Spreadsheet.vi"("file path (dialog if empty)"=w171, "format (%.3f)"="%e", "1D data"=w146, "append to file? (new file:F)"=TRUE, "error in (no error)"=w176, "transpose? (no:F)"=w149) -> ("new file path (Not A Path if cancelled)"=w172:path, "error out"=w173:errorcluster)  [unwired: 8 in]
    n71 = Divide(x=w159, y=w157) -> (x/y=w156:dbl)
    n72 = Add(x=w156, y="Relative threshold") -> (x+y=w139:dbl)
    "Threshold" <- w139
    n73 = call-poly <vilib>:"Write Delimited Spreadsheet.vi"("file path (dialog if empty)"=w172, "format (%.3f)"="%e", "1D data"=w143, "append to file? (new file:F)"=TRUE, "error in (no error)"=w173, "transpose? (no:F)"=w149) -> ("error out"=w152:errorcluster)  [unwired: 8 in, 1 out]
    n74 = To Fixed-Point(fixed-point type=fxp<+,16,4> 0.0 ("AI Trigger Configuration.Hystesis Value"), number=w139) -> (fixed-point=w154:fxp<+,16,4>)
    n75 = flat-sequence {
      tunnel: w154 -> [w216]
      tunnel: w152 -> [w217]
      tunnel: [w217] -> w134
      tunnel: [w221] -> w151
      tunnel: w134 -> [w221]
      tunnel: [w220] -> w133
      frame #0 {
        n76 = Multiply(x=w216, y=fxp<+,16,4> 0.0) -> (x*y=w214:fxp<+,32,8>)
        n77 = local read "Ic parameters"() -> (w219:T2)
        n78 = To Fixed-Point(fixed-point type=fxp<+,16,4> 0.0 ("AI Trigger Configuration.Hystesis Value"), number=w214) -> (fixed-point=w215:fxp<+,16,4>)
        n79 = Bundle By Name(cluster=w219, "AI Trigger Configuration.Trigger Level"=w216, "AI Trigger Configuration.Hystesis Value"=w215) -> (w218:T2)
        n80 = local write "Ic parameters"(w218) -> ()
      }
      frame #1 {
        n81 = local read "Ic parameters"() -> (w220:T2)
      }
    }
    n82 = Unbundle By Name(w133) -> ("Records Num"=w194:i32, "Record Samples"=w193:u32)
    n83 = while {
      tunnel: w205 -> [w243]
      tunnel: w151 -> [w242]
      tunnel: [w240] -> w204
      tunnel: [w239] -> w203
      stop <- w241 stop-if-true
      n84 = property class="Network Stream Endpoint"(reference=w243, error in=w242) -> (reference out=w240:refnum<k21>, error out=w239:errorcluster, "AvailElmntsForWrite"=w245:i32)
      n85 = Equal?(x=w245, y=1) -> (x = y?=w241:bool)
    }
    n86 = To Long Integer(number=w193) -> (32bit integer=w180:i32)
    n87 = Multiply(x=w194, y=w180) -> (x*y=w192:i32)
    n88 = shared-variable-write(w204, w203, w133) -> (w197:refnum<k21>, w201:errorcluster)  [unwired: 1 in, 1 out]
    n89 = for {
      N: w192 -> [_]
      tunnel: w202 -> [w238]
      tunnel: w201 -> [w237]
      tunnel: [w236] -> w166
      tunnel: [w235] -> w200
      tunnel: [w234] -> w198 mode=indexing
      n90 = call "network stream read.vi"("error in (no error)"=w237, "endpoint in"=w238) -> ("error out"=w236:errorcluster, "Data"=w234:fxp<+/-,17,5>, "endpoint out"=w235:refnum<k21>)  [unwired: 7 in]
    }
    n91 = To Double Precision Float(number=w198) -> (double precision float=w164:dbl[])
    n92 = for {
      tunnel: w164 -> [w223] mode=indexing
      tunnel: w180 -> [w229]
      shift-right: [w225] -> w142
      shift-left: dbl[] [] -> [w224]
      i -> [w228]
      n93 = Quotient & Remainder(x=w228, y=w229) -> (x-y*floor(x/y)=w227:i32)  [unwired: 1 out]
      n94 = Equal?(x=1, y=w227) -> (x = y?=w222:bool)
      n95 = case shown="False" w222 {
        tunnel: [w230 w233] -> w225
        tunnel: w224 -> [w230 w232]
        tunnel: w223 -> [_ w231]
        frame False {
        }
        frame True {
          n96 = Build Array (concatenate)(w232, w231) -> (w233:dbl[])
        }
      }
    }
    n97 = local read "Current Scale factor"() -> (w140:dbl)
    n98 = Multiply(x=w142, y=w140) -> (x*y=w141:dbl[])
    n99 = call <vilib>:"Histogram.vi"("intervals"=100, "X"=w141) -> ("Histogram Graph"=→"Histogram Graph":T3)  [unwired: 6 in, 3 out]
    n100 = call-poly <vilib>:"Write Delimited Spreadsheet.vi"("file path (dialog if empty)"=w163, "format (%.3f)"="%e", "1D data"=w141, "append to file? (new file:F)"=TRUE, "error in (no error)"=w166, "transpose? (no:F)"=FALSE) -> ("error out"=w165:errorcluster)  [unwired: 8 in, 1 out]
    "Current Field mT" <- w136
  }
  n101 = Destroy Stream Endpoint(8:w63, 11:w66) -> (0:w76:errorcluster)
  n102 = Destroy Stream Endpoint(8:w76, 11:w67) -> (0:w69:errorcluster)
  n103 = Destroy Stream Endpoint(8:w69, 11:w64) -> (0:w17:errorcluster)
  n104 = local read "Magnet Device Select"() -> (w15:string)
  n105 = call "set single axis Field Module.vi"("Magnet Device Select"=w15, "error in (no error)"=w17, "Init"=FALSE, "Field Target mT"=0.0, "Exec"=w11, "Field Rate mT per sec"=1.0, "final"=w11) -> ("error out"=w16:errorcluster)  [unwired: 12 in]
  n106 = shared-variable "NI-cRIO-9063-01bc8cc6\\network varibles.lvlib\\RT Stop"(TRUE ("RT Stop"), error in=w16) -> (error out=w2:errorcluster)
  n107 = call "Stop cRIO fast measure.vi"("error in (no error)"=w2, "VI reference"=w3, "application reference"=w4) -> ("error out"=→"error out":errorcluster)  [unwired: 8 in]
